vi "Initialise TDMS.vi"(8 "error in (no error)":errorcluster) -> (0 "error out":errorcluster, 3 "tdms file out":refnum<k34>)   [LabVIEW 2017]
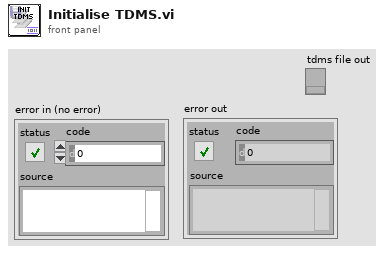
[diagram p1: front panel]
types:
  T1 = enum16{"open", "open or create", "create or replace", "create", "open (read-only)"}
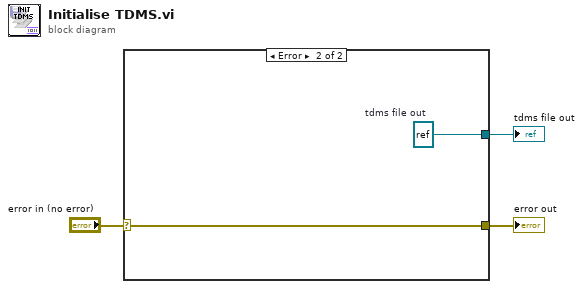
[diagram p0: block diagram]
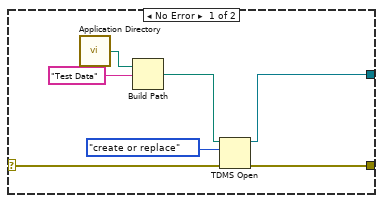
[diagram p2: hidden frame]
diagram:
  n1 = case shown="Error" "error in (no error)" {
    selector: "error in (no error)" -> [w6 w11]
    tunnel: [w5 w11] -> w2
    tunnel: [w4 w12] -> w1
    frame No Error {
      n2 = call <vilib>:"Application Directory.vi"() -> ("Application Directory"=w7:path)
      n3 = Build Path(base path=w7, name or relative path="Test Data") -> (appended path=w9:path)
      n4 = TDMS Open(8:w6, 10:T1."create or replace" ("operation (0:open)"), 11:w9) -> (0:w5:errorcluster, 3:w4:refnum<k34>)  [unwired: 4 in]
    }
    frame Error {
      w12 = refnum<k34> refnum  # tdms file out
    }
  }
  "error out" <- w2
  "tdms file out" <- w1
